vi "Test S7 API.vi"() -> ()   [LabVIEW 2020]
doc: "S7 API Tester."
uses:
  S7.lvlib
panel:
  in  "Show Block Diagram":bool
  in  "Stop Module":bool
  in  "Start Module":bool
  in  "Hide Module Panel":bool
  in  "Show Module Panel":bool
  out "Status":string
  out "Module Running?":bool
  # "This VI tests the API for the Module."
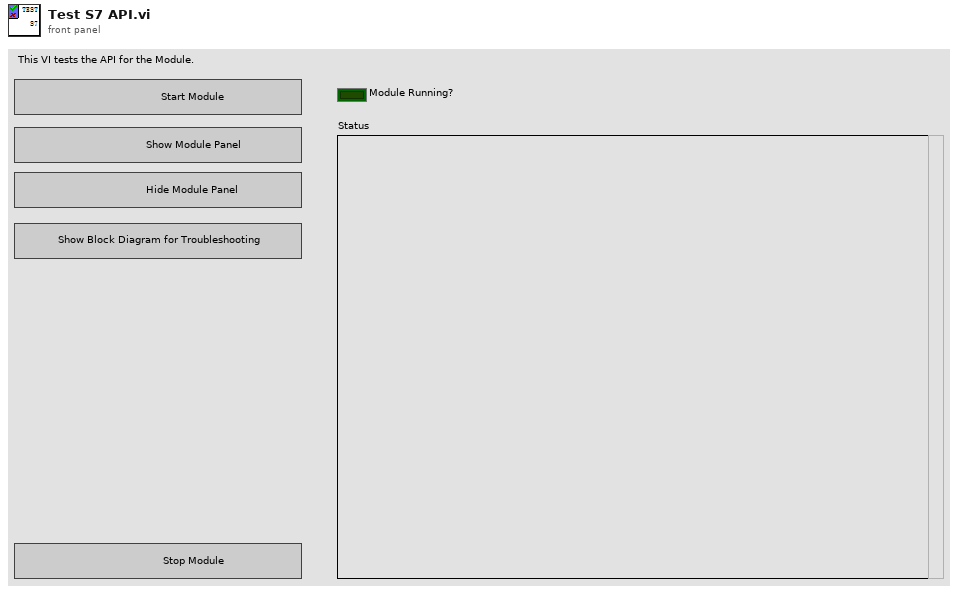
[diagram p1: front panel]
types:
  T1 = typedef "S7.lvlib/Broadcast Events--cluster.ctl" = cluster{"Module Did Init":refnum<user-event>, "Status Updated":refnum<user-event>, "Error Reported":refnum<user-event>, "Module Did Stop":refnum<user-event>, "Update Module Execution Status":refnum<user-event>}
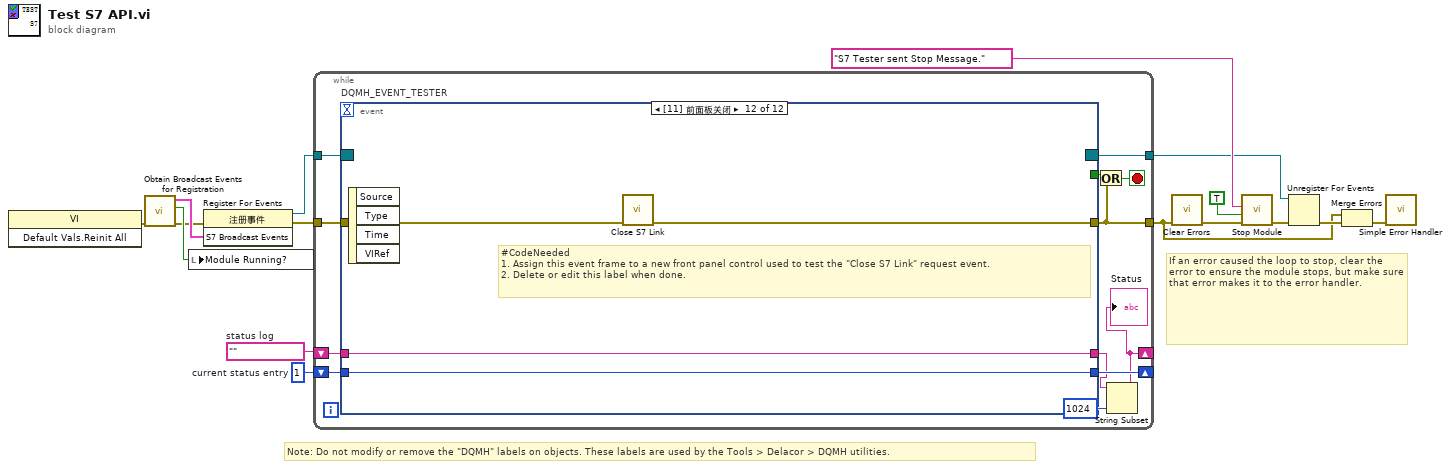
[diagram p0: block diagram]
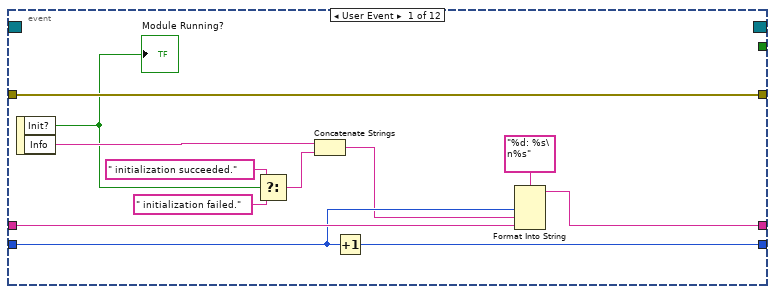
[diagram p2: hidden frame]
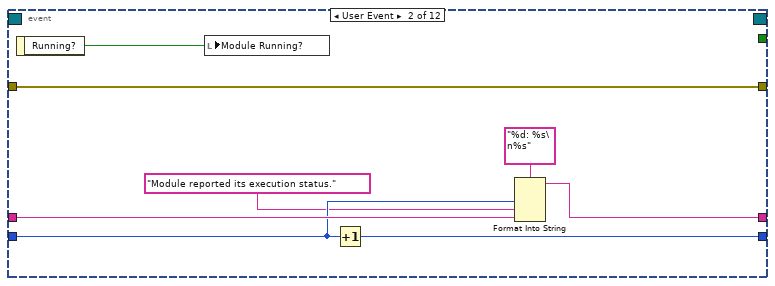
[diagram p3: hidden frame]
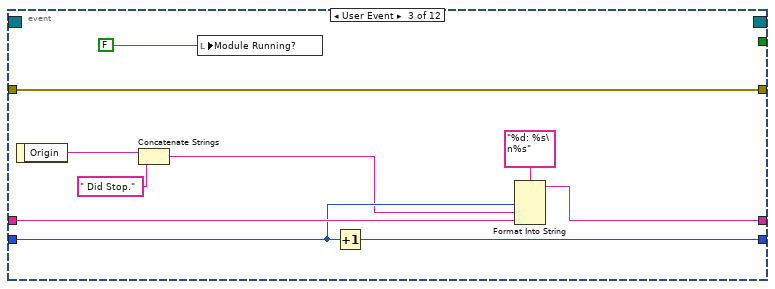
[diagram p4: hidden frame]
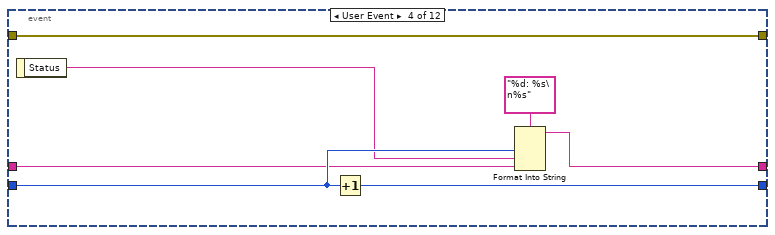
[diagram p5: hidden frame]
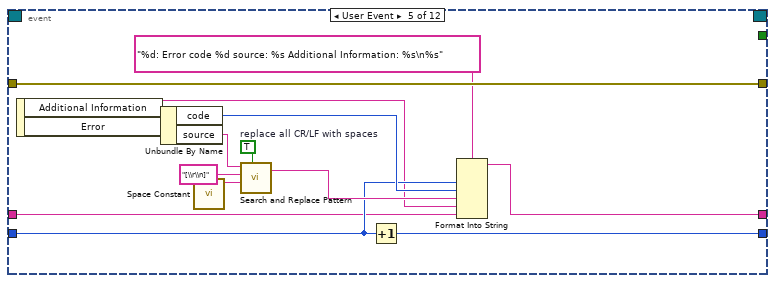
[diagram p6: hidden frame]
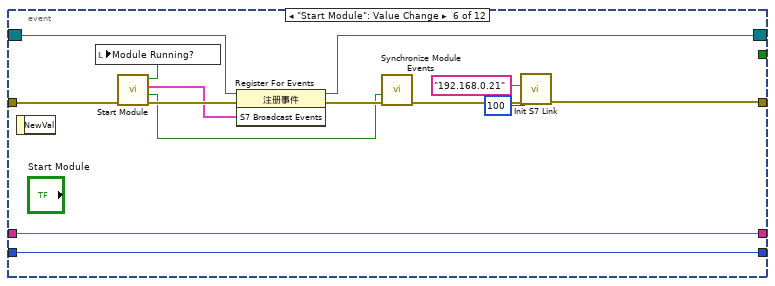
[diagram p7: hidden frame]
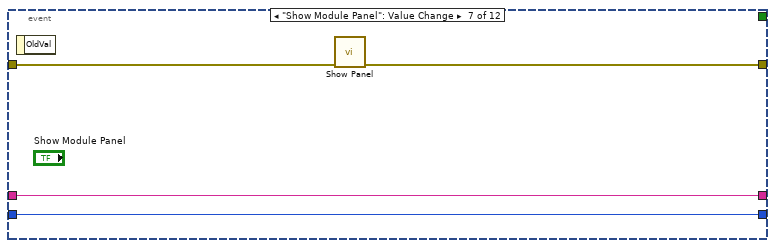
[diagram p8: hidden frame]
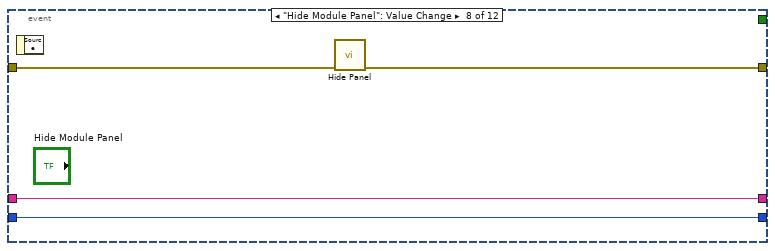
[diagram p9: hidden frame]
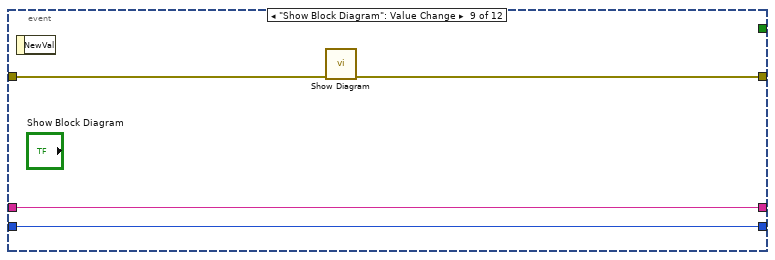
[diagram p10: hidden frame]
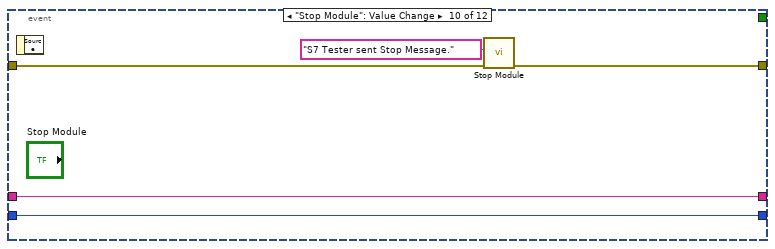
[diagram p11: hidden frame]
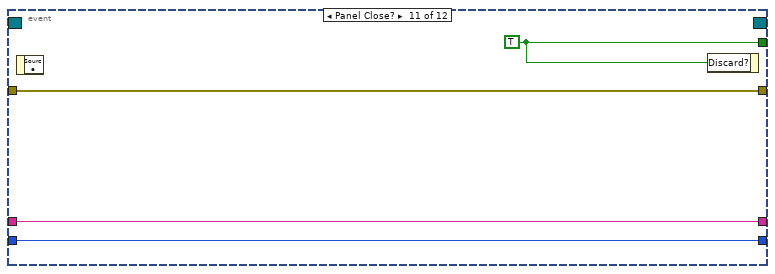
[diagram p12: hidden frame]
diagram:
  w12 = 1  # current status entry
  w13 = ""  # status log
  # "If an error caused the loop to stop, clear the error to ensure the module stops, but make sure that error makes it to the error handler."
  # "Note: Do not modify or remove the \"DQMH\" labels on objects. These labels are used by the Tools > Delacor > DQMH utilities."
  n1 = invoke class="VI" method="Default Vals.Reinit All"() -> (error out=w2:errorcluster)  [unwired: 3 in, 2 out]
  n2 = call "Obtain Broadcast Events for Registration.vi"("error in (no error)"=w2) -> ("error out"=w1:errorcluster, "Already running?"=w3:bool, "S7 Broadcast Events"=w10:T1)  [unwired: 8 in]
  n3 = local write "Module Running?"(w3) -> ()
  n4 = register-events(error in=w1, w10) -> (reference out=w9:refnum<event-registration>, error out=w11:errorcluster)  [unwired: 1 in]
  n5 = while {
    tunnel: w9 -> [w28]
    tunnel: [w20] -> w4
    shift-right: [w17] -> _
    shift-left: w13 -> [w25]
    shift-right: [w24] -> _
    shift-left: w12 -> [w26]
    tunnel: w11 -> [w22]
    tunnel: [w21] -> w8
    stop <- w23 stop-if-true
    n6 = event "DQMH_EVENT_TESTER" shown="[11] 前面板关闭" {
      selector: w28 -> [_ _ _ _ _ w87 _ _ _ _ _ _]
      dyn-events: [_ _ _ _ _ w86 _ _ _ _ _ _] -> w21
      timeout: _ -> [_ _ _ _ _ _ _ _ _ _ _ _]
      tunnel: [_ _ _ _ _ _ _ _ _ _ w114 _] -> w27
      tunnel: [w40 w42 w49 w59 w79 w82 w97 w101 w102 w108 w111 w115] -> w20
      tunnel: w26 -> [w37 w46 w56 w62 w69 w90 w95 w99 w103 w109 w112 w116]
      tunnel: w25 -> [w38 w47 w57 w61 w67 w91 w96 w100 w104 w110 w113 w117]
      tunnel: [w35 w44 w54 w63 w70 w91 w96 w100 w104 w110 w113 w117] -> w19
      tunnel: [w36 w45 w55 w65 w68 w90 w95 w99 w103 w109 w112 w116] -> w24
      tunnel: w22 -> [w40 w42 w49 w59 w79 w85 w94 w98 w105 w106 w111 w118]
      event User Event {
        n7 = event-data() -> ("Init?"=w32:bool, "Info"=w34:string)  [unwired: 1 in]
        "Module Running?" <- w32
        n8 = Select(t=" initialization succeeded.", s=w32, f=" initialization failed.") -> (s? t:f=w29:string)
        n9 = Concatenate Strings(w34, w29) -> (w33:string)
        n10 = Increment(x=w37) -> (x+1=w36:i32)
        n11 = Format Into String(format string="%d: %s\n%s", w37, w33, w38) -> (resulting string=w35:string)  [unwired: 2 in, 1 out]
      }
      event User Event {
        n12 = event-data() -> ("Running?"=w41:bool)  [unwired: 1 in]
        n13 = local write "Module Running?"(w41) -> ()
        n14 = Increment(x=w46) -> (x+1=w45:i32)
        n15 = Format Into String(format string="%d: %s\n%s", w46, "Module reported its execution status.", w47) -> (resulting string=w44:string)  [unwired: 2 in, 1 out]
      }
      event User Event {
        n16 = event-data() -> ("Origin"=w53:string)  [unwired: 1 in]
        n17 = Concatenate Strings(w53, " Did Stop.") -> (w52:string)
        n18 = local write "Module Running?"(FALSE ("Module Did Init?")) -> ()
        n19 = Increment(x=w56) -> (x+1=w55:i32)
        n20 = Format Into String(format string="%d: %s\n%s", w56, w52, w57) -> (resulting string=w54:string)  [unwired: 2 in, 1 out]
      }
      event User Event {
        n21 = event-data() -> ("Status"=w60:string)  [unwired: 1 in]
        n22 = Increment(x=w62) -> (x+1=w65:i32)
        n23 = Format Into String(format string="%d: %s\n%s", w62, w60, w61) -> (resulting string=w63:string)  [unwired: 2 in, 1 out]
      }
      event User Event {
        w75 = TRUE  # replace all CR/LF with spaces
        n24 = event-data() -> ("Additional Information"=w66:string, "Error"=w71:errorcluster)  [unwired: 1 in]
        n25 = Unbundle By Name(w71) -> ("code"=w72:i32, "source"=w73:string)
        n26 = call <vilib>:"Space Constant.vi"() -> ("String"=w76:string)
        n27 = call <vilib>:"Search and Replace Pattern.vi"("string"=w73, "regular expression (\"\")"="[\\r\\n]" ("regular expression (\"\")"), "replace string (\"\")"=w76, "replace all? (F)"=w75) -> ("result string"=w74:string)  [unwired: 1 in, 1 out]
        n28 = Increment(x=w69) -> (x+1=w68:i32)
        n29 = Format Into String(format string="%d: Error code %d source: %s Additional Information: %s\n%s", w69, w72, w74, w66, w67) -> (resulting string=w70:string)  [unwired: 2 in, 1 out]
      }
      event "Start Module": Value Change {
        n30 = event-data() -> ()  [unwired: 1 in, 1 out]
        n31 = call "Start Module.vi"("error in (no error)"=w85) -> ("error out"=w92:errorcluster, "Wait for Event Sync?"=w89:bool, "S7 Broadcast Events"=w88:T1, "Module Was Already Running?"=w84:bool)  [unwired: 7 in]
        n32 = local write "Module Running?"(w84) -> ()
        n33 = register-events(reference=w87, error in=w92, w88) -> (reference out=w86:refnum<event-registration>, error out=w93:errorcluster)
        n34 = call "Synchronize Module Events.vi"("error in (no error)"=w93, "Wait for Event Sync?"=w89) -> ("error out"=w83:errorcluster)  [unwired: 9 in]
        n35 = call "Init S7 Link.vi"("error in (no error)"=w83, "超时"=100, "IP"="192.168.0.21") -> ("error out"=w82:errorcluster)  [unwired: 8 in]
      }
      event "Show Module Panel": Value Change {
        n36 = event-data() -> ()  [unwired: 1 in, 1 out]
        n37 = call "Show Panel.vi"("error in (no error)"=w94) -> ("error out"=w97:errorcluster)  [unwired: 10 in]
      }
      event "Hide Module Panel": Value Change {
        n38 = event-data() -> ()  [unwired: 1 in, 1 out]
        n39 = call "Hide Panel.vi"("error in (no error)"=w98) -> ("error out"=w101:errorcluster)  [unwired: 10 in]
      }
      event "Show Block Diagram": Value Change {
        n40 = event-data() -> ()  [unwired: 1 in, 1 out]
        n41 = call "Show Diagram.vi"("error in (no error)"=w105) -> ("error out"=w102:errorcluster)  [unwired: 10 in]
      }
      event "Stop Module": Value Change {
        n42 = event-data() -> ()  [unwired: 1 in, 1 out]
        n43 = call "Stop Module.vi"("error in (no error)"=w106, "Origin"="S7 Tester sent Stop Message.") -> ("error out"=w108:errorcluster)  [unwired: 9 in]
      }
      event Panel Close? {
        w114 = TRUE ("Discard?")
        n44 = event-data() -> ()  [unwired: 1 in, 1 out]
        n45 = event-data("Discard?"=w114) -> ()  [unwired: 1 in, 1 out]
      }
      event Panel Close {
        # "#CodeNeeded\n1. Assign this event frame to a new front panel control used to test the \"Close S7 Link\" request event.\n2. Delete or edit this label when done."
        n46 = event-data() -> ()  [unwired: 1 in, 4 out]
        n47 = call "Close S7 Link.vi"("error in (no error)"=w118) -> ("error out"=w115:errorcluster)  [unwired: 10 in]
      }
    }
    n48 = Or(x=w27, y=w20) -> (x .or. y?=w23:bool)
    n49 = String Subset(string=w19, length (rest)=1024 ("长度（剩余）")) -> (substring=w17:string)  [unwired: 1 in]
    "Status" <- w17
  }
  n50 = call <vilib>:"Clear Errors.vi"("error in (no error)"=w4) -> ("error out"=w6:errorcluster)  [unwired: 5 in, 1 out]
  n51 = call "Stop Module.vi"("error in (no error)"=w6, "Wait for Module to Stop? (F)"=TRUE ("Wait for Module to stop?"), "Origin"="S7 Tester sent Stop Message.") -> ("error out"=w15:errorcluster)  [unwired: 8 in]
  n52 = Unregister For Events(event registration refnum=w8, error in=w15) -> (error out=w16:errorcluster)
  n53 = Merge Errors(w4, w16) -> (w5:errorcluster)
  n54 = call <vilib>:"Simple Error Handler.vi"("error in (no error)"=w5) -> ()  [unwired: 4 in, 5 out]
